vi "Actor Core.vi"(8 "error in":errorcluster, 11 "Root Panel Actor in":refnum<class "Root Panel Actor.lvclass">) -> (0 "error out":errorcluster, 3 "Actor out":refnum<class "Actor.lvclass">)   [LabVIEW 2021, in "Root Panel.lvlib" / "Root Panel Actor.lvclass"]
doc: "The user interface for this panel.\n\n----\nPlease see the following web address for additional documentation and tutorial information:\nhttp://www.mooregoodideas.com/mgi-panel-manager/\n\nAuthor: Derek Trepanier\n\nCopyright (c) 2018, Moore Good Ideas, Inc.\n\nAll rights reserved.\n\nRedistribution and use in source and binary forms, with or without modification, are permitted provided that the following conditions are met:\n\n * Redistributions of source code must retain the above copyright notice, this list of conditions and the following disclaimer.\n * Redistributions in binary form must reproduce the above copyright notice, this list of conditions and the following disclaimer in the documentation and/or other materials provided with the distribution.\n * Neither the name of Moore Good Ideas, Inc. nor the names of its contributors may be used to endorse or promote products derived from this software without specific prior written permission.\n\nTHIS SOFTWARE IS PROVIDED BY THE COPYRIGHT HOLDERS AND CONTRIBUTORS \"AS IS\" AND ANY EXPRESS OR IMPLIED WARRANTIES, INCLUDING, BUT NOT LIMITED TO, THE IMPLIED WARRANTIES OF MERCHANTABILITY AND FITNESS FOR A PARTICULAR PURPOSE ARE DISCLAIMED. IN NO EVENT SHALL THE COPYRIGHT OWNER OR CONTRIBUTORS BE LIABLE FOR ANY DIRECT, INDIRECT, INCIDENTAL, SPECIAL, EXEMPLARY, OR CONSEQUENTIAL DAMAGES (INCLUDING, BUT NOT LIMITED TO, PROCUREMENT OF SUBSTITUTE GOODS OR SERVICES; LOSS OF USE, DATA, OR PROFITS; OR BUSINESS INTERRUPTION) HOWEVER CAUSED AND ON ANY THEORY OF LIABILITY, WHETHER IN CONTRACT, STRICT LIABILITY, OR TORT (INCLUDING NEGLIGENCE OR OTHERWISE) ARISING IN ANY WAY OUT OF THE USE OF THIS SOFTWARE, EVEN IF ADVISED OF THE POSSIBILITY OF SUCH DAMAGE."
uses:
  Root Panel Actor.lvclass
  C:/Program Files (x86)/National Instruments/LabVIEW 2021/vi.lib/MGI/Panel Manager/Panel Actor/Panel Actor/Panel Actor.lvclass
  <vilib>/ActorFramework/Actor/Actor.lvclass
  Root Panel Actor.lvclass/Root Panel Actor.ctl
  <vilib>/ActorFramework/Message Enqueuer/Message Enqueuer.lvclass/Message Enqueuer.ctl
  <vilib>/ActorFramework/Message Enqueuer/Enqueue.vi
  <vilib>/ActorFramework/Stop Msg/Stop Msg.lvclass
  C:/Program Files (x86)/National Instruments/LabVIEW 2021/vi.lib/ActorFramework/Message/Message.lvclass
  <vilib>/ActorFramework/Message Priority Queue/Priority Enqueue.vi
  Appearance Actor/Appearance Actor/Appearance Actor.lvclass
  <vilib>/MGI/Panel Manager/Panel Actor/Panel Actor/Panel Actor.lvclass
  Windows/System32/user32.dll
  <vilib>/MGI/Panel Manager/Panel Actor/Panel Actor Messages/Show Panel Msg/Show Panel Msg.lvclass
panel:
  in  "Title Bar L":bool
  out "App Icon":picture
  in  "Title Bar M":bool
  out "Title":string
  in  "Maximize":bool
  in  "Close":bool
  in  "Minimize":bool
  in  "Title Bar R":bool
  in  "Settings":bool
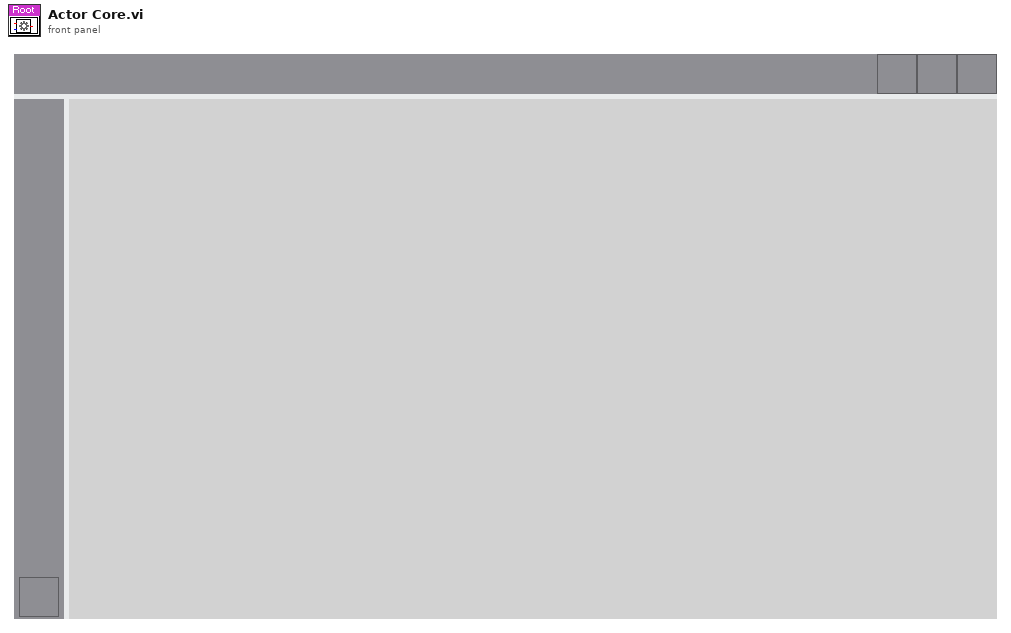
[diagram p1: front panel]
types:
  T1 = cluster{"left":i16, "top":i16, "right":i16, "bottom":i16}
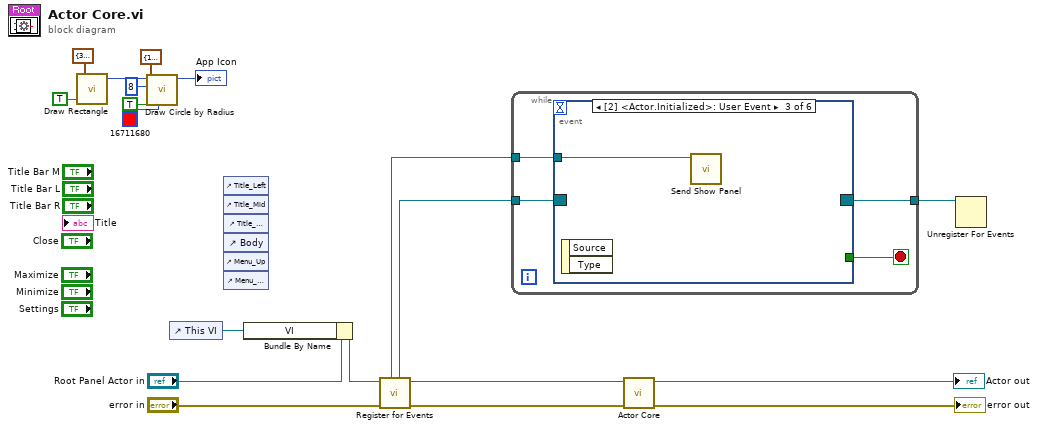
[diagram p0: block diagram]
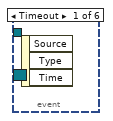
[diagram p2: hidden frame]
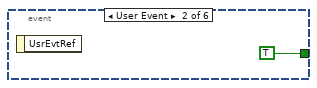
[diagram p3: hidden frame]
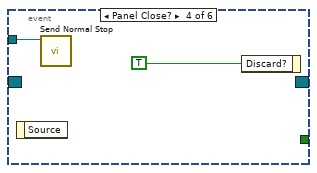
[diagram p4: hidden frame]
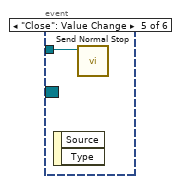
[diagram p5: hidden frame]
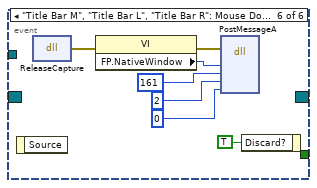
[diagram p6: hidden frame]
diagram:
  n1 = call <vilib>:"Draw Rectangle.vi"("rect"=T1 {"left"=3, "top"=3, "right"=40, "bottom"=30}, "fill?(F)"=TRUE) -> ("new picture"=w7:picture)  [unwired: 7 in]
  n2 = call <vilib>:"Draw Circle by Radius.vi"("color(black)"=u32 16711680, "fill?(F)"=TRUE, "pixel center"=cluster{"horizontal":i16, "vertical":i16} {"horizontal"=15, "vertical"=12}, "radius"=i16 8, "picture"=w7) -> ("new picture"=→"App Icon":picture)  [unwired: 6 in]
  n3 = control-ref of="This VI"() -> (w12:refnum<vi>)
  n4 = control-ref of="Title_Left"() -> ()  [unwired: 1 out]
  n5 = control-ref of="Title_Mid"() -> ()  [unwired: 1 out]
  n6 = control-ref of="Title_Right"() -> ()  [unwired: 1 out]
  n7 = control-ref of="Body"() -> ()  [unwired: 1 out]
  n8 = control-ref of="Menu_Up"() -> ()  [unwired: 1 out]
  n9 = control-ref of="Menu_Down"() -> ()  [unwired: 1 out]
  n10 = Bundle By Name(cluster="Root Panel Actor in", "VI"=w12) -> (w13:refnum<class "Root Panel Actor.lvclass">)
  n11 = call <vilib>:"Register for Events.vi"("Error In"="error in", "Panel Actor in"=w13) -> ("Error Out"=w10:errorcluster, "Panel Actor out"=w1:refnum<class "Root Panel Actor.lvclass">, "Pnl Actor"=w14:refnum<event-registration>, "Self Enqueuer"=w15:refnum<class "Message Enqueuer.lvclass">)  [unwired: 6 in]
  n12 = while {
    tunnel: w14 -> [w23]
    tunnel: w15 -> [w22]
    tunnel: [w20] -> w16
    stop <- w21 stop-if-true
    n13 = event shown="[2] <Actor.Initialized>: User Event" {
      selector: w23 -> [_ _ _ _ _ _]
      dyn-events: [_ _ _ _ _ _] -> w20
      timeout: _ -> [_ _ _ _ _ _]
      tunnel: w22 -> [_ _ w25 w27 w28 _]
      tunnel: [_ TRUE _ _ _ _] -> w21
      event Timeout {
        n14 = event-data() -> ()  [unwired: 1 in, 3 out]
      }
      event User Event {
        n15 = event-data() -> ()  [unwired: 1 in, 1 out]
      }
      event User Event {
        n16 = event-data() -> ()  [unwired: 1 in, 2 out]
        n17 = call <vilib>:"Send Show Panel.vi"("Message Enqueuer in"=w25) -> ()  [unwired: 9 in, 2 out]
      }
      event Panel Close? {
        n18 = event-data() -> ()  [unwired: 1 in, 1 out]
        n19 = call <vilib>:"Send Normal Stop.vi"("Message Enqueuer"=w27) -> ()  [unwired: 10 in, 1 out]
        n20 = event-data("Discard?"=TRUE) -> ()  [unwired: 1 in, 1 out]
      }
      event "Close": Value Change {
        n21 = event-data() -> ()  [unwired: 1 in, 2 out]
        n22 = call <vilib>:"Send Normal Stop.vi"("Message Enqueuer"=w28) -> ()  [unwired: 10 in, 1 out]
      }
      event "Title Bar M", "Title Bar L", "Title Bar R": Mouse Down? {
        n23 = event-data() -> ()  [unwired: 1 in, 1 out]
        n24 = dll-call lib="C:/Windows/System32/user32.dll" fn="ReleaseCapture"() -> (error out=w34:errorcluster)  [unwired: 4 in, 1 out]
        n25 = property class="VI"(error in=w34) -> (error out=w33:errorcluster, "FP.NativeWindow"=w32:u64)  [unwired: 1 in, 1 out]
        n26 = dll-call lib="C:/Windows/System32/user32.dll" fn="PostMessageA"(error in=w33, "arg1"=w32, "arg2"=161, "arg3"=2, "arg4"=0) -> ()  [unwired: 7 in, 2 out]
        n27 = event-data("Discard?"=TRUE) -> ()  [unwired: 1 in, 1 out]
      }
    }
  }
  n28 = call-parent "Actor Core.vi"("error in"=w10, "Panel Actor in"=w1) -> ("error out"=→"error out":errorcluster, "Actor out"=→"Actor out":refnum<class "Actor.lvclass">)  [unwired: 8 in]
  n29 = Unregister For Events(event registration refnum=w16) -> ()  [unwired: 1 in, 1 out]
